vi "Edit Search Panel.vi"(8 "error in (no error)":errorcluster, 11 "BetterSearch in":refnum<class "BetterSearch.lvclass">) -> ()   [LabVIEW 2020, in "Better Search.lvlib" / "BetterSearch.lvclass"]
uses:
  BetterSearch.lvclass
  Search/Search.lvclass
  Data Types/Search Scope.ctl
  BetterSearch.lvclass/BetterSearch.ctl
  Data Types/Search Params.ctl
  Data Types/Search Type.ctl
  Data Types/Scope Options.ctl
  Better Search.lvlib
panel:
  out "Exclude Label":string="Match In:"
  in  "instr.lib":bool
  in  "user.lib":bool
  in  "vi.lib":bool
  in  "Dependencies":bool
  in  "Add All Targets":bool
  out "Selected Targets":i32(listbox)
  out "Member Index":i32
  out "Type ID":string
  out "Starting VI":string
  in  "Start":bool
  out "Targets":refnum<vi>[](array[refnum])
  in  "Scope":T1
  in  "Search Type":T2(tab)
  in  "String Value":bool
  in  "Text":string caption="Search Text"
  in  "Include Labels":bool
  in  "Include Captions":bool
  in  "Include Node Name":bool
  out "Match Label":string="Match In:"
  out "Member Name":string
  in  "Type Name":string
  in  "Member Access":bool
  in  "Member Write":bool
  in  "Member Read":bool
  in  "Specify Member":bool
  out "Current Search":refnum<class "Search.lvclass">
  # "Double-click a target to remove it from the list."
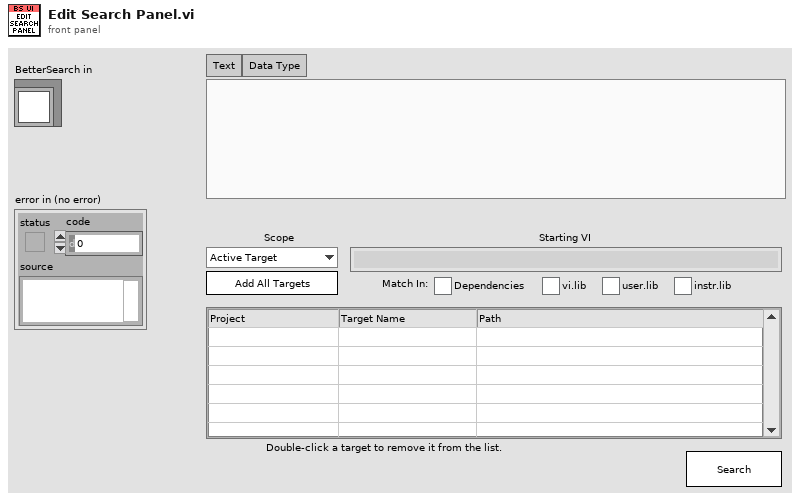
[diagram p1: front panel]
types:
  T1 = typedef "Better Search.lvlib/Search Scope.ctl" = enum16{"Active Target", "Active Project", "Specific Targets", "Active VI", "Active Hierarchy"}
  T2 = enum32{"General", "Text", "Data Type", "VI", "Node"}
  T3 = typedef "Better Search.lvlib/BetterSearch.lvclass/Edit Events.ctl" = cluster{"New Edit":refnum<user-event>, "Close Edit Panel":refnum<user-event>}
  T4 = typedef "Better Search.lvlib/Search Params.ctl" = cluster{"Type":T5, "Type ID":string, "Text":string, "Scope":T1, "Targets":refnum<vi>[], "Scope Options":T6, "Typedef Path":path, "Member Graph Index":i32, "Member TypeID":string}
  T5 = typedef "Better Search.lvlib/Search Type.ctl" = enum16{"Generic", "Text", "Data Type", "VI", "Node"}
  T6 = typedef "Better Search.lvlib/Scope Options.ctl" = cluster{"Include Labels":bool, "Include Captions":bool, "Include Node Name":bool, "Member Access":bool, "Member Read":bool, "Member Write":bool, "Member Name":string, "String Value":bool, "Dependencies":bool, "vi.lib":bool, "user.lib":bool, "instr.lib":bool}
  T7 = enum8{"Enabled", "Disabled", "Disabled and Grayed Out"}
  T8 = typedef "Better Search.lvlib/Search Context.ctl" = cluster{"Type ID":string, "VI Refnum":refnum<vi>, "Starting Text":string, "Shift?":bool, "App Ref":refnum<vi>, "Start Search Type":T9, "Item Graph":T10[], "Variant":variant}
  T9 = typedef "Better Search.lvlib/Start Search Type.ctl" = enum16{"Auto", "Text", "Data Type", "Bundle"}
  T10 = typedef "Better Search.lvlib/Type Reflection Item.ctl" = cluster{"Parent":i32, "Depth":i32, "Children":i32[], "Skip":bool, "Name":string, "Type":variant, "TypeID":string}
  T11 = typedef "Better Search.lvlib/BetterSearch.lvclass/Search Validation Failure.ctl" = enum16{"None", "Empty Text"}
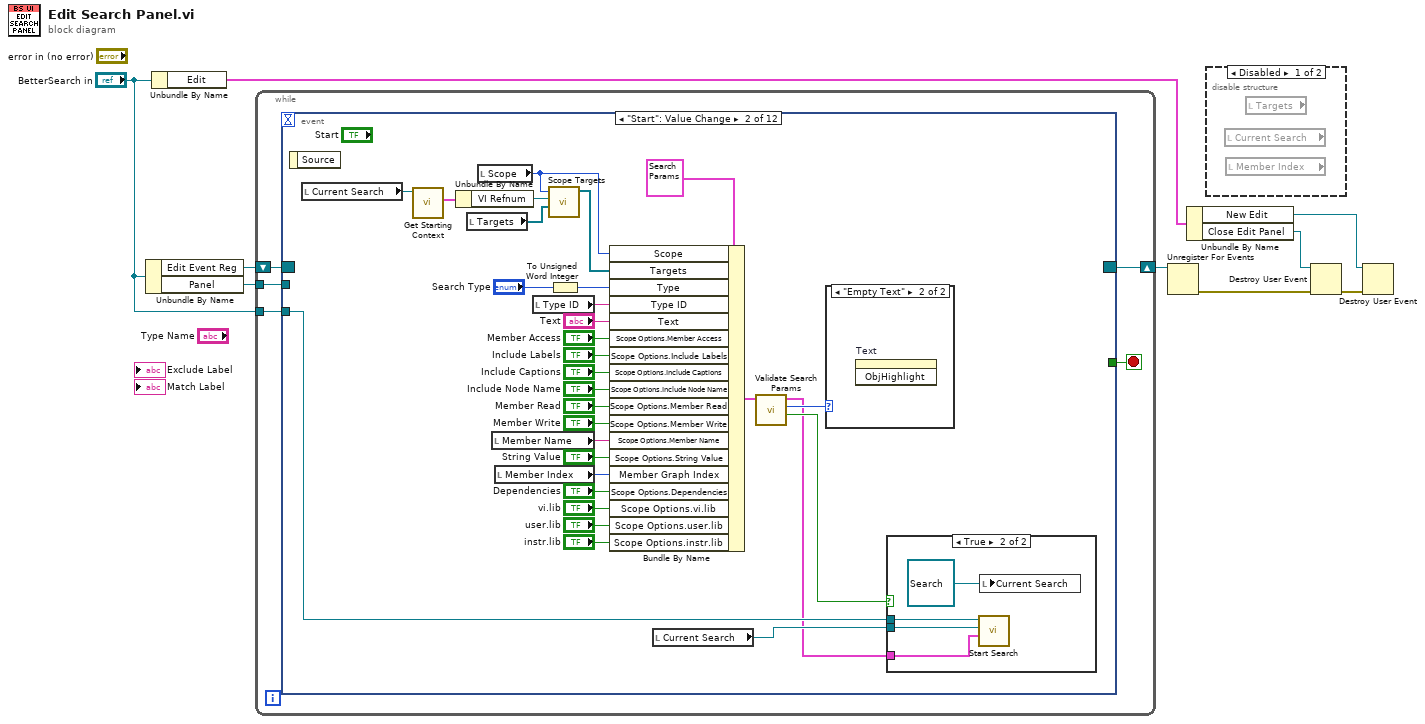
[diagram p0: block diagram]
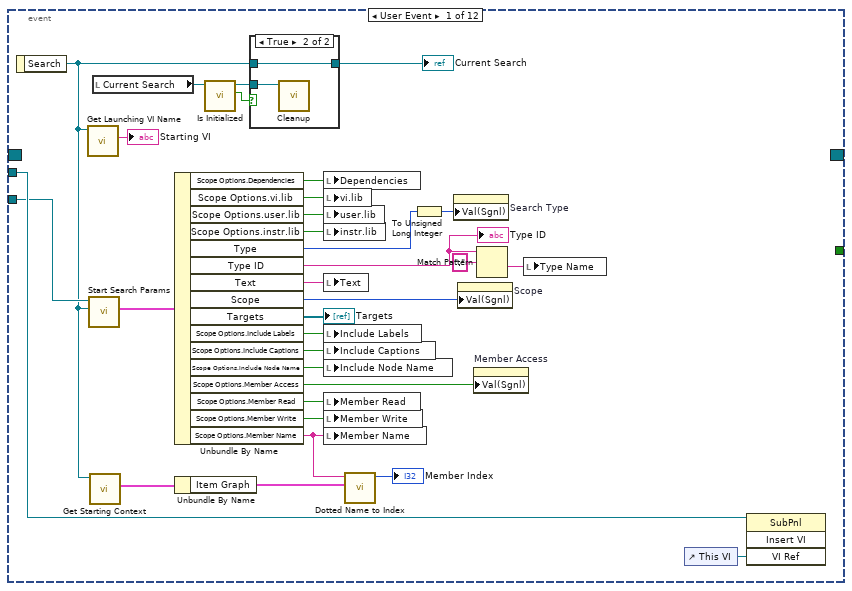
[diagram p3: hidden frame]
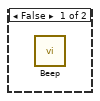
[diagram p6: hidden frame]
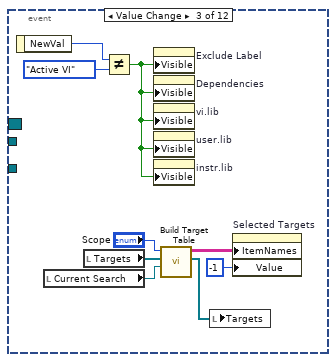
[diagram p7: hidden frame]
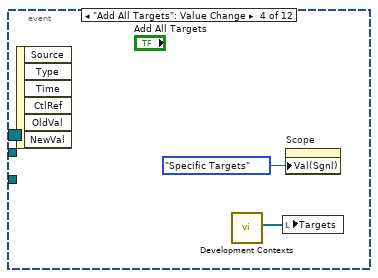
[diagram p8: hidden frame]
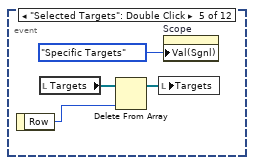
[diagram p9: hidden frame]
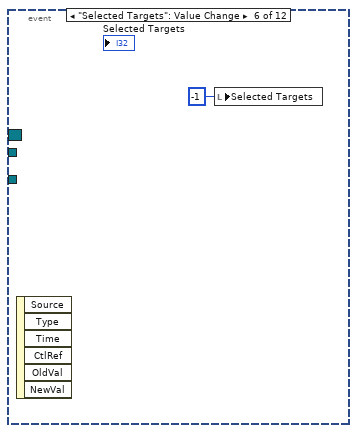
[diagram p10: hidden frame]
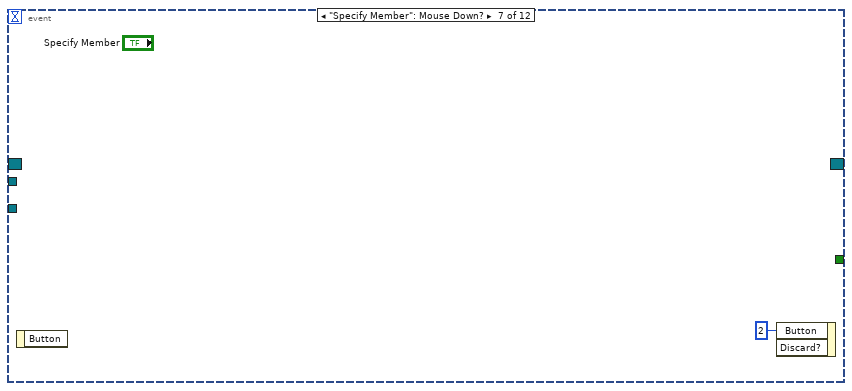
[diagram p11: hidden frame]
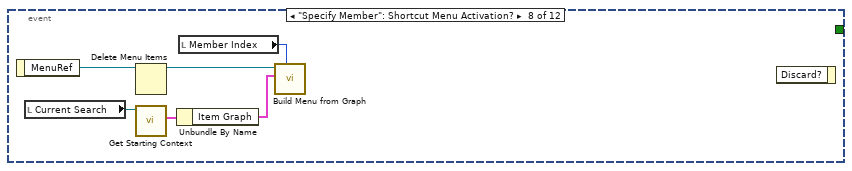
[diagram p12: hidden frame]
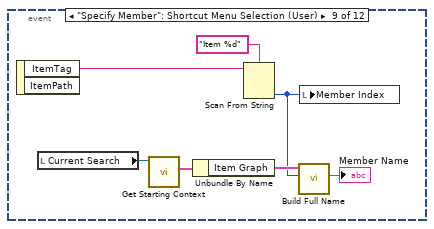
[diagram p13: hidden frame]
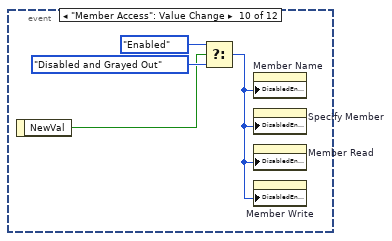
[diagram p14: hidden frame]
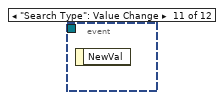
[diagram p15: hidden frame]
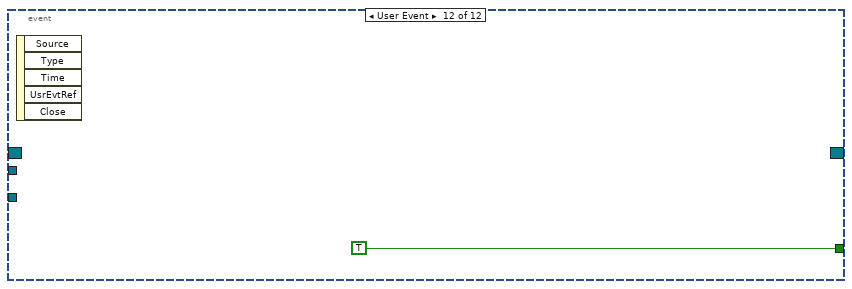
[diagram p16: hidden frame]
diagram:
  n1 = Unbundle By Name("BetterSearch in") -> ("Edit Event Reg"=w8:refnum<event-registration>, "Panel"=w2:refnum<vi>)
  n2 = Unbundle By Name("BetterSearch in") -> ("Edit"=w6:T3)
  n3 = while {
    shift-right: [w13] -> w9
    shift-left: w8 -> [w14]
    tunnel: w2 -> [w11]
    tunnel: "BetterSearch in" -> [w10]
    stop <- w12 stop-if-true
    n4 = event shown="[1] \"Start\": Value Change" {
      selector: w14 -> [_ _ _ _ _ _ _ _ _ _ _ _]
      dyn-events: [_ _ _ _ _ _ _ _ _ _ _ _] -> w13
      timeout: _ -> [_ _ _ _ _ _ _ _ _ _ _ _]
      tunnel: [_ _ _ _ _ _ _ _ _ _ _ TRUE] -> w12
      tunnel: w11 -> [w46 _ _ _ _ _ _ _ _ _ _ _]
      tunnel: w10 -> [w37 w79 _ _ _ _ _ _ _ _ _ _]
      event User Event {
        n5 = event-data() -> ("Search"=w20:refnum<class "Search.lvclass">)  [unwired: 1 in]
        n6 = call "Get Launching VI Name.vi"("Search in"=w20) -> ("Launching VI Name"=→"Starting VI":string)  [unwired: 8 in, 2 out]
        n7 = call "Start Search Params.vi"("Search in"=w20, "BetterSearch in"=w37) -> ("Start Params"=w44:T4)  [unwired: 7 in, 2 out]
        n8 = call "Get Starting Context.vi"("Search in"=w20) -> ("Starting Context"=w27:T8)  [unwired: 8 in, 2 out]
        n9 = local read "Current Search"() -> (w23:refnum<class "Search.lvclass">)
        n10 = Unbundle By Name(w44) -> ("Scope Options.Dependencies"=w15:bool, "Scope Options.vi.lib"=w16:bool, "Scope Options.user.lib"=w17:bool, "Scope Options.instr.lib"=w18:bool, "Type"=w36:T5, "Type ID"=w32:string, "Text"=w35:string, "Scope"=w24:T1, "Targets"=→"Targets":refnum<vi>[], "Scope Options.Include Labels"=w38:bool, "Scope Options.Include Captions"=w39:bool, "Scope Options.Include Node Name"=w40:bool, "Scope Options.Member Access"=w29:bool, "Scope Options.Member Read"=w33:bool, "Scope Options.Member Write"=w34:bool, "Scope Options.Member Name"=w28:string)
        "Type ID" <- w32
        n11 = Unbundle By Name(w27) -> ("Item Graph"=w26:T10[])
        n12 = call "Is Initialized.vi"("Search in"=w23) -> ("Initialized"=w22:bool, "Search out"=w21:refnum<class "Search.lvclass">)  [unwired: 8 in, 1 out]
        n13 = case shown="True" w22 {
          tunnel: w21 -> [_ w48]
          tunnel: w20 -> [w47 w49]
          tunnel: [w47 w49] -> w19
          frame False {
          }
          frame True {
            n14 = call "Cleanup.vi"("Search in"=w48) -> ()  [unwired: 10 in, 1 out]
          }
        }
        "Current Search" <- w19
        n15 = local write "Dependencies"(w15) -> ()
        n16 = local write "vi.lib"(w16) -> ()
        n17 = local write "user.lib"(w17) -> ()
        n18 = local write "instr.lib"(w18) -> ()
        n19 = local write "Text"(w35) -> ()
        n20 = local write "Include Labels"(w38) -> ()
        n21 = local write "Include Captions"(w39) -> ()
        n22 = local write "Include Node Name"(w40) -> ()
        n23 = local write "Member Read"(w33) -> ()
        n24 = local write "Member Write"(w34) -> ()
        n25 = local write "Member Name"(w28) -> ()
        n26 = call "Dotted Name to Index.vi"("Item Graph"=w26, "Dotted Name"=w28) -> ("Index"=→"Member Index":i32)  [unwired: 9 in]
        n27 = To Unsigned Long Integer(number=w36) -> (unsigned 32bit integer=w42:u32)
        n28 = property on="Search Type" class="TabCtl (strict)"("Val(Sgnl)"=w42) -> ()  [unwired: 2 in, 2 out]
        n29 = property on="Scope" class="Enum (strict)"("Val(Sgnl)"=w24) -> ()  [unwired: 2 in, 2 out]
        n30 = property on="Member Access" class="Bool (strict)"("Val(Sgnl)"=w29) -> ()  [unwired: 2 in, 2 out]
        n31 = Match Pattern(string=w32, regular expression=":") -> (after substring=w30:string)  [unwired: 1 in, 3 out]
        n32 = local write "Type Name"(w30) -> ()
        n33 = control-ref of="This VI"() -> (w45:refnum<vi>)
        n34 = invoke class="SubPnl" method="Insert VI"(reference=w46, "VI Ref"=w45) -> ()  [unwired: 2 in, 4 out]
      }
      event "Start": Value Change {
        n35 = event-data() -> ()  [unwired: 1 in, 1 out]
        n36 = local read "Current Search"() -> (w62:refnum<class "Search.lvclass">)
        n37 = call "Get Starting Context.vi"("Search in"=w62) -> ("Starting Context"=w61:T8)  [unwired: 8 in, 2 out]
        n38 = Unbundle By Name(w61) -> ("VI Refnum"=w60:refnum<vi>)
        n39 = local read "Targets"() -> (w59:refnum<vi>[])
        n40 = local read "Scope"() -> (w58:T1)
        n41 = local read "Member Name"() -> (w65:string)
        n42 = local read "Member Index"() -> (w56:i32)
        n43 = local read "Type ID"() -> (w74:string)
        n44 = call "Scope Targets.vi"("Specific Targets"=w59, "Launching VI"=w60, "Search Scope"=w58) -> ("Scope Targets"=w57:refnum<vi>[])  [unwired: 8 in]
        n45 = To Unsigned Word Integer(number="Search Type") -> (unsigned 16bit integer=w75:u16)
        n46 = Bundle By Name(cluster=T4 {"Type"=enum."Generic", "Type ID"="", "Text"="", "Scope"=enum."Active Target", "Targets"=[], "Scope Options"={"Include Labels"=FALSE, "Include Captions"=FALSE, "Include Node Name"=FALSE, "Member Access"=FALSE, "Member Read"=FALSE, "Member Write"=FALSE, "Member Name"="", "String Value"=FALSE, "Dependencies"=FALSE, "vi.lib"=FALSE, "user.lib"=FALSE, "instr.lib"=FALSE}, "Typedef Path"=path "", "Member Graph Index"=0, "Member TypeID"=""} ("Search Params"), "Scope"=w58, "Targets"=w57, "Type"=w75, "Type ID"=w74, "Text"="Text", "Scope Options.Member Access"="Member Access", "Scope Options.Include Labels"="Include Labels", "Scope Options.Include Captions"="Include Captions", "Scope Options.Include Node Name"="Include Node Name", "Scope Options.Member Read"="Member Read", "Scope Options.Member Write"="Member Write", "Scope Options.Member Name"=w65, "Scope Options.String Value"="String Value", "Member Graph Index"=w56, "Scope Options.Dependencies"="Dependencies", "Scope Options.vi.lib"="vi.lib", "Scope Options.user.lib"="user.lib", "Scope Options.instr.lib"="instr.lib") -> (w70:T4)
        n47 = local read "Current Search"() -> (w63:refnum<class "Search.lvclass">)
        n48 = call "Validate Search Params.vi"("Search Params In"=w70) -> ("Valid?"=w69:bool, "Search Validation Failure"=w51:T11, "Search Params"=w50:T4)  [unwired: 8 in]
        n49 = case shown="\"Empty Text\"" w51 {
          frame "None" {
          }
          frame "Empty Text" {
            n50 = invoke on="Text" class="Str" method="ObjHighlight"() -> ()  [unwired: 3 in, 3 out]
          }
        }
        n51 = case shown="True" w69 {
          tunnel: w79 -> [_ w83]
          tunnel: w50 -> [_ w82]
          tunnel: w63 -> [_ w81]
          frame False {
            n52 = call <vilib>:"Beep.vi"() -> ()  [unwired: 12 in]
          }
          frame True {
            n53 = call "Start Search.vi"("Search Params"=w82, "Search"=w81, "BetterSearch in"=w83) -> ()  [unwired: 7 in, 2 out]
            n54 = local write "Current Search"(refnum<class "Search.lvclass"> refnum ("Current Search")) -> ()
          }
        }
      }
      event Value Change {
        n55 = event-data() -> ("NewVal"=w86:T1)  [unwired: 1 in]
        n56 = local read "Current Search"() -> (w90:refnum<class "Search.lvclass">)
        n57 = local read "Targets"() -> (w91:refnum<vi>[])
        n58 = Not Equal?(x=w86, y=Search_Scope."Active VI") -> (x != y?=w84:bool)
        n59 = property on="Exclude Label" class="Str"("Visible"=w84) -> ()  [unwired: 2 in, 2 out]
        n60 = property on="Dependencies" class="Bool (strict)"("Visible"=w84) -> ()  [unwired: 2 in, 2 out]
        n61 = property on="vi.lib" class="Bool (strict)"("Visible"=w84) -> ()  [unwired: 2 in, 2 out]
        n62 = property on="user.lib" class="Bool (strict)"("Visible"=w84) -> ()  [unwired: 2 in, 2 out]
        n63 = property on="instr.lib" class="Bool (strict)"("Visible"=w84) -> ()  [unwired: 2 in, 2 out]
        n64 = call "Build Target Table.vi"("Search"=w90, "Targets In"=w91, "Scope"="Scope") -> ("Targets"=w88:refnum<vi>[], "Target Table"=w89:string[][])  [unwired: 7 in]
        n65 = local write "Targets"(w88) -> ()
        n66 = property on="Selected Targets" class="MCListbox (strict)"("ItemNames"=w89, "Value"=-1 ("Selected Targets")) -> ()  [unwired: 2 in, 2 out]
      }
      event "Add All Targets": Value Change {
        n67 = event-data() -> ()  [unwired: 1 in, 6 out]
        n68 = call "Development Contexts.vi"() -> ("Development Contexts"=w94:refnum<vi>[])  [unwired: 11 in]
        n69 = local write "Targets"(w94) -> ()
        n70 = property on="Scope" class="Enum (strict)"("Val(Sgnl)"=Search_Scope."Specific Targets" ("Scope")) -> ()  [unwired: 2 in, 2 out]
      }
      event "Selected Targets": Double Click {
        n71 = event-data() -> ("Row"=w97:i32)  [unwired: 1 in]
        n72 = local read "Targets"() -> (w98:refnum<vi>[])
        n73 = Delete From Array(array=w98, index=w97) -> (array with subset deleted=w96:refnum<vi>[])  [unwired: 1 in, 1 out]
        n74 = local write "Targets"(w96) -> ()
        n75 = property on="Scope" class="Enum (strict)"("Val(Sgnl)"=Search_Scope."Specific Targets" ("Value (Signaling)")) -> ()  [unwired: 2 in, 2 out]
      }
      event "Selected Targets": Value Change {
        n76 = event-data() -> ()  [unwired: 1 in, 6 out]
        n77 = local write "Selected Targets"(-1 ("Selected Targets")) -> ()
      }
      event "Specify Member": Mouse Down? {
        n78 = event-data() -> ()  [unwired: 1 in, 1 out]
        n79 = event-data("Button"=u16 2) -> ()  [unwired: 2 in, 1 out]
      }
      event "Specify Member": Shortcut Menu Activation? {
        n80 = event-data() -> ("MenuRef"=w102:refnum<k9>)  [unwired: 1 in]
        n81 = local read "Current Search"() -> (w106:refnum<class "Search.lvclass">)
        n82 = Delete Menu Items(9:w102) -> (3:w101:refnum<k9>)  [unwired: 3 in, 1 out]
        n83 = call "Get Starting Context.vi"("Search in"=w106) -> ("Starting Context"=w105:T8)  [unwired: 8 in, 2 out]
        n84 = Unbundle By Name(w105) -> ("Item Graph"=w104:T10[])
        n85 = local read "Member Index"() -> (w103:i32)
        n86 = call "Build Menu from Graph.vi"("Selection"=w103, "Items"=w104, "Menu"=w101) -> ()  [unwired: 9 in]
        n87 = event-data() -> ()  [unwired: 2 in, 1 out]
      }
      event "Specify Member": Shortcut Menu Selection (User) {
        n88 = event-data() -> ("ItemTag"=w113:string)  [unwired: 1 in, 1 out]
        n89 = local read "Current Search"() -> (w111:refnum<class "Search.lvclass">)
        n90 = call "Get Starting Context.vi"("Search in"=w111) -> ("Starting Context"=w110:T8)  [unwired: 8 in, 2 out]
        n91 = Unbundle By Name(w110) -> ("Item Graph"=w109:T10[])
        n92 = Scan From String(format string="Item %d", input string=w113) -> (output 1=w108:i32)  [unwired: 3 in, 3 out]
        n93 = call "Build Full Name.vi"("Index"=w108, "Item Graph In"=w109) -> ("Name"=→"Member Name":string)  [unwired: 8 in, 1 out]
        n94 = local write "Member Index"(w108) -> ()
      }
      event "Member Access": Value Change {
        n95 = event-data() -> ("NewVal"=w115:bool)  [unwired: 1 in]
        n96 = Select(t=T7."Enabled" ("Disabled"), s=w115, f=T7."Disabled and Grayed Out") -> (s? t:f=w114:T7)
        n97 = property on="Member Name" class="Str"("DisabledEnum"=w114) -> ()  [unwired: 2 in, 2 out]
        n98 = property on="Specify Member" class="Bool"("DisabledEnum"=w114) -> ()  [unwired: 2 in, 2 out]
        n99 = property on="Member Read" class="Bool (strict)"("DisabledEnum"=w114) -> ()  [unwired: 2 in, 2 out]
        n100 = property on="Member Write" class="Bool (strict)"("DisabledEnum"=w114) -> ()  [unwired: 2 in, 2 out]
      }
      event "Search Type": Value Change {
        n101 = event-data() -> ()  [unwired: 1 in, 1 out]
      }
      event User Event {
        n102 = event-data() -> ()  [unwired: 1 in, 5 out]
      }
    }
  }
  n103 = Unregister For Events(event registration refnum=w9) -> (error out=w7:errorcluster)  [unwired: 1 in]
  n104 = Unbundle By Name(w6) -> ("New Edit"=w3:refnum<user-event>, "Close Edit Panel"=w5:refnum<user-event>)
  n105 = disable-structure shown="Disabled" {
    frame Disabled {
      n106 = local read "Current Search"() -> ()  [unwired: 1 out]
      n107 = local read "Member Index"() -> ()  [unwired: 1 out]
      n108 = local read "Targets"() -> ()  [unwired: 1 out]
    }
    frame Enabled {
    }
  }
  n109 = Destroy User Event(user event=w5, error in=w7) -> (error out=w4:errorcluster)
  n110 = Destroy User Event(user event=w3, error in=w4) -> ()  [unwired: 1 out]
